vi "Single IV and Ic distribution v2.vi"() -> ()   [LabVIEW 2024]
uses:
  <vilib>/LabVIEW Targets/FPGA/cRIO/shared/nicrio_ModuleControls/nicrio_cRIO-9775_RecordDataRates4ChansRing.ctl
  RT fast data.ctl
  <vilib>/LabVIEW Targets/FPGA/cRIO/shared/nicrio_ModuleControls/nicrio_BasicConversionTime.ctl
  Ramps.ctl
  cRIO VI parameters.vi
  <resource>/objmgr/ni.dex.rc
  <vilib>/Analysis/NI_AALBase.lvlib
panel:
  in  "Tab Control 3":enum32{"Distribution", "IV"}(tab)
  out "Histogram Graph":T1(graph)={"X Values"=[3.702567138671875, 3.708775634765625, 3.714984130859375, 3.7211926269531252, 3.7274011230468753, 3.7336096191406254, 3.7398181152343755, 3.7460266113281255, 3.7522351074218756, 3.7584436035156257, 3.7646520996093757, 3.770860595703126, 3.777069091796876, 3.783277587890626, 3.789486083984376, 3.795694580078126, 3.801903076171876, 3.8081115722656262, 3.8143200683593763, 3.8205285644531264, 3.8267370605468765, 3.8329455566406265, 3.8391540527343766, 3.8453625488281267, 3.8515710449218767, 3.857779541015627, 3.863988037109377, 3.870196533203127, 3.876405029296877, 3.882613525390627, 3.888822021484377, 3.8950305175781272, 3.9012390136718773, 3.9074475097656274, 3.9136560058593775, 3.9198645019531275, 3.9260729980468776, 3.9322814941406277, 3.9384899902343777, 3.944698486328128, 3.950906982421878, 3.957115478515628, 3.963323974609378, 3.969532470703128, 3.975740966796878, 3.9819494628906282, 3.9881579589843783, 3.9943664550781284, 4.0005749511718784, 4.0067834472656285, 4.012991943359379, 4.019200439453129, 4.025408935546879, 4.031617431640629, 4.037825927734379, 4.044034423828129, 4.050242919921879, 4.056451416015629, 4.062659912109379, 4.068868408203129, 4.075076904296879, 4.081285400390629, 4.087493896484379, 4.0937023925781295, 4.09991088867188, 4.10611938476563, 4.11232788085938, 4.11853637695313, 4.12474487304688, 4.13095336914063, 4.13716186523438, 4.14337036132813, 4.14957885742188, 4.15578735351563, 4.16199584960938, 4.16820434570313, 4.17441284179688, 4.1806213378906305, 4.186829833984381, 4.193038330078131, 4.199246826171881, 4.205455322265631, 4.211663818359381, 4.217872314453131, 4.224080810546881, 4.230289306640631, 4.236497802734381, 4.242706298828131, 4.248914794921881, 4.255123291015631, 4.261331787109381, 4.2675402832031315, 4.273748779296882, 4.279957275390632, 4.286165771484382, 4.292374267578132, 4.298582763671882, 4.304791259765632, 4.310999755859382, 4.317208251953132], "Histogram: h(x)"=[1, 0, 0, 0, 1, 1, 0, 3, 2, 4, 3, 2, 1, 5, 10, 11, 14, 19, 24, 21, 32, 20, 49, 60, 74, 75, 110, 85, 117, 114, 161, 127, 186, 168, 225, 211, 265, 245, 280, 241, 355, 309, 353, 285, 369, 286, 349, 271, 355, 304, 277, 301, 252, 286, 218, 288, 193, 251, 165, 214, 135, 154, 132, 137, 101, 120, 75, 86, 58, 75, 49, 45, 25, 29, 25, 12, 20, 11, 9, 13, 5, 6, 4, 7, 2, 6, 1, 2, 1, 0, 1, 2, 1, 1, 0, 0, 0, 0, 1, 1]}
  out "Array":dbl[](array[numeric])
  out "Start time ms":u32=3399600001
  out "Time to Init ms":u32=668
  out "Threshold":dbl=0.23218066406250001
  out "IV Curve":cluster{"X":dbl[], "Y":dbl[]}[](graph)
  in  "length":i32=3300
  in  "Begin index":i32
  out "I data":dbl[](array[numeric])
  in  "Tab Control":T2(tab)
  in  "Data folder":path=path "C:/Users/gyue/Desktop/GA01_202401"
  in  "Sample Name":string
  out "output file name":string="20240127-224058-Single IV and Dist_Dist.dat"
  in  "IV Record Samples":u32=4300
  in  "Dist Records Num":i32=10000
  in  "IV Record Data Rate":T3=200 items=["20.000 MS/s (NI 9775)"=1, "10.00 MS/s (NI 9775)"=2, "6.667 MS/s (NI 9775)"=3, "5.000 MS/s (NI 9775)"=4, "2.500 MS/s (NI 9775)"=8, "1.667 MS/s (NI 9775)"=12, "1.250 MS/s (NI 9775)"=16, "1.000 MS/s (NI 9775)"=20, "833.333 KS/s (NI 9775)"=24, "714.286 KS/s (NI 9775)"=28, "625.000 KS/s (NI 9775)"=32, "555.556 KS/s (NI 9775)"=36, "500.000 KS/s (NI 9775)"=40, "454.545 KS/s (NI 9775)"=44, "416.667 KS/s (NI 9775)"=48, "384.615 KS/s (NI 9775)"=52, "357.143 KS/s (NI 9775)"=56, "333.333 KS/s (NI 9775)"=60, "312.500 KS/s (NI 9775)"=64, "294.118 KS/s (NI 9775)"=68, "277.778 KS/s (NI 9775)"=72, "263.158 KS/s (NI 9775)"=76, "250.000 KS/s (NI 9775)"=80, "238.095 KS/s (NI 9775)"=84, "227.273 KS/s (NI 9775)"=88, "217.391 KS/s (NI 9775)"=92, "208.333 KS/s (NI 9775)"=96, "200.000 KS/s (NI 9775)"=100, "192.308 KS/s (NI 9775)"=104, "185.185 KS/s (NI 9775)"=108, "178.571 KS/s (NI 9775)"=112, "172.414 KS/s (NI 9775)"=116, "166.667 KS/s (NI 9775)"=120, "161.290 KS/s (NI 9775)"=124, "156.250 KS/s (NI 9775)"=128, "151.515 KS/s (NI 9775)"=132, "147.059 KS/s (NI 9775)"=136, "142.857 KS/s (NI 9775)"=140, "138.889 KS/s (NI 9775)"=144, "135.135 KS/s (NI 9775)"=148, "131.579 KS/s (NI 9775)"=152, "128.205 KS/s (NI 9775)"=156, "125.000 KS/s (NI 9775)"=160, "121.951 KS/s (NI 9775)"=164, "119.048 KS/s (NI 9775)"=168, "116.279 KS/s (NI 9775)"=172, "113.636 KS/s (NI 9775)"=176, "111.111 KS/s (NI 9775)"=180, "108.696 KS/s (NI 9775)"=184, "106.383 KS/s (NI 9775)"=188, "104.167 KS/s (NI 9775)"=192, "102.041 KS/s (NI 9775)"=196, "100.000 KS/s (NI 9775)"=200, "50.000 KS/s (NI 9775)"=400, "33.333 KS/s (NI 9775)"=600, "25.000 KS/s (NI 9775)"=800, "20.000 KS/s (NI 9775)"=1000, "16.667 KS/s (NI 9775)"=1200, "14.286 KS/s (NI 9775)"=1400, "12.500 KS/s (NI 9775)"=1600, "11.111 KS/s (NI 9775)"=1800, "10.000 KS/s (NI 9775)"=2000, "9.091 KS/s (NI 9775)"=2200, "8.333 KS/s (NI 9775)"=2400, "7.692 KS/s (NI 9775)"=2600, "7.143 KS/s (NI 9775)"=2800, "6.667 KS/s (NI 9775)"=3000, "6.250 KS/s (NI 9775)"=3200, "5.882 KS/s (NI 9775)"=3400, "5.556 KS/s (NI 9775)"=3600, "5.000 KS/s (NI 9775)"=4000, "4.762 KS/s (NI 9775)"=4200, "4.545 KS/s (NI 9775)"=4400, "4.348 KS/s (NI 9775)"=4600, "4.167 KS/s (NI 9775)"=4800, "4.000 KS/s (NI 9775)"=5000, "3.846 KS/s (NI 9775)"=5200, "3.571 KS/s (NI 9775)"=5600, "3.333 KS/s (NI 9775)"=6000, "3.125 KS/s (NI 9775)"=6400, "2.941 KS/s (NI 9775)"=6800, "2.778 KS/s (NI 9775)"=7200, "2.632 KS/s (NI 9775)"=7600, "2.500 KS/s (NI 9775)"=8000, "2.381 KS/s (NI 9775)"=8400, "2.273 KS/s (NI 9775)"=8800, "2.174 KS/s (NI 9775)"=9200, "2.083 KS/s (NI 9775)"=9600, "2.000 KS/s (NI 9775)"=10000, "1.923 KS/s (NI 9775)"=10400, "1.852 KS/s (NI 9775)"=10800, "1.786 KS/s (NI 9775)"=11200, "1.724 KS/s (NI 9775)"=11600, "1.667 KS/s (NI 9775)"=12000, "1.613 KS/s (NI 9775)"=12400, "1.563 KS/s (NI 9775)"=12800, "1.515 KS/s (NI 9775)"=13200, "1.471 KS/s (NI 9775)"=13600, "1.429 KS/s (NI 9775)"=14000, "1.389 KS/s (NI 9775)"=14400, "1.351 KS/s (NI 9775)"=14800, "1.316 KS/s (NI 9775)"=15200, "1.282 KS/s (NI 9775)"=15600, "1.250 KS/s (NI 9775)"=16000, "1.220 KS/s (NI 9775)"=16400, "1.190 KS/s (NI 9775)"=16800, "1.163 KS/s (NI 9775)"=17200, "1.136 KS/s (NI 9775)"=17600, "1.111 KS/s (NI 9775)"=18000, "1.087 KS/s (NI 9775)"=18400, "1.064 KS/s (NI 9775)"=18800, "1.042 KS/s (NI 9775)"=19200, "1.020 KS/s (NI 9775)"=19600, "1.000 KS/s (NI 9775)"=20000, "0.980 KS/s (NI 9775)"=20400, "0.962 KS/s (NI 9775)"=20800, "0.943 KS/s (NI 9775)"=21200, "0.926 KS/s (NI 9775)"=21600, "0.909 KS/s (NI 9775)"=22000, "0.893 KS/s (NI 9775)"=22400, "0.877 KS/s (NI 9775)"=22800, "0.862 KS/s (NI 9775)"=23200, "0.847 KS/s (NI 9775)"=23600, "0.833 KS/s (NI 9775)"=24000, "0.820 KS/s (NI 9775)"=24400, "0.806 KS/s (NI 9775)"=24800, "0.794 KS/s (NI 9775)"=25200, "0.781 KS/s (NI 9775)"=25600, "0.694 KS/s (NI 9775)"=28800, "0.625 KS/s (NI 9775)"=32000, "0.568 KS/s (NI 9775)"=35200, "0.521 KS/s (NI 9775)"=38400, "0.446 KS/s (NI 9775)"=44800, "0.391 KS/s (NI 9775)"=51200, "0.347 KS/s (NI 9775)"=57600, "0.313 KS/s (NI 9775)"=64000]
  in  "Current Scale factor":dbl=1.0
  in  "Voltage Scale factor":dbl=0.0001
  in  "Relative Threshold":dbl=0.2
  in  "Read point":i32=1
  in  "Wire resistance":dbl
  in  "Zero avg":i32=1000
  in  "Ic Wait before trigger us":u32=30000
  in  "Ic Cutoff delay usec":u32
  in  "Trigger Slope":u16(ring) items=["Positive", "Negative"]
  in  "Tab Control 2":enum32{"IV parameters", "Ic parameters"}(tab)
  out "IV parameters":T4={"Records Num"=1, "AI Trigger Configuration"={"Trigger Slope"=enum."Positive", "Trigger Level"=0.10009765625, "Hystesis Value"=0.094970703125, "AI Channel"=0}, "Record PreTrigger Samples"=1, "Record Samples"=4300, "Ic Cut off or curve"=FALSE, "Record Data Rate"=200, "Wait before trigger us"=0, "Cutoff delay usec"=0, "Timing Mode"=enum."High Resolution", "Trigger length ticks"=1, "Timeout"=-1, "Ramps"={"Amp"=8.0, "Delay time 10us"=3000, "Ramp1 time 10us"=1000, "Ramp2 time 10us"=200, "Ramp3 time 10us"=100, "End time 10us"=0}} {"Record Data Rate" items=["20.000 MS/s (NI 9775)"=1, "10.00 MS/s (NI 9775)"=2, "6.667 MS/s (NI 9775)"=3, "5.000 MS/s (NI 9775)"=4, "2.500 MS/s (NI 9775)"=8, "1.667 MS/s (NI 9775)"=12, "1.250 MS/s (NI 9775)"=16, "1.000 MS/s (NI 9775)"=20, "833.333 KS/s (NI 9775)"=24, "714.286 KS/s (NI 9775)"=28, "625.000 KS/s (NI 9775)"=32, "555.556 KS/s (NI 9775)"=36, "500.000 KS/s (NI 9775)"=40, "454.545 KS/s (NI 9775)"=44, "416.667 KS/s (NI 9775)"=48, "384.615 KS/s (NI 9775)"=52, "357.143 KS/s (NI 9775)"=56, "333.333 KS/s (NI 9775)"=60, "312.500 KS/s (NI 9775)"=64, "294.118 KS/s (NI 9775)"=68, "277.778 KS/s (NI 9775)"=72, "263.158 KS/s (NI 9775)"=76, "250.000 KS/s (NI 9775)"=80, "238.095 KS/s (NI 9775)"=84, "227.273 KS/s (NI 9775)"=88, "217.391 KS/s (NI 9775)"=92, "208.333 KS/s (NI 9775)"=96, "200.000 KS/s (NI 9775)"=100, "192.308 KS/s (NI 9775)"=104, "185.185 KS/s (NI 9775)"=108, "178.571 KS/s (NI 9775)"=112, "172.414 KS/s (NI 9775)"=116, "166.667 KS/s (NI 9775)"=120, "161.290 KS/s (NI 9775)"=124, "156.250 KS/s (NI 9775)"=128, "151.515 KS/s (NI 9775)"=132, "147.059 KS/s (NI 9775)"=136, "142.857 KS/s (NI 9775)"=140, "138.889 KS/s (NI 9775)"=144, "135.135 KS/s (NI 9775)"=148, "131.579 KS/s (NI 9775)"=152, "128.205 KS/s (NI 9775)"=156, "125.000 KS/s (NI 9775)"=160, "121.951 KS/s (NI 9775)"=164, "119.048 KS/s (NI 9775)"=168, "116.279 KS/s (NI 9775)"=172, "113.636 KS/s (NI 9775)"=176, "111.111 KS/s (NI 9775)"=180, "108.696 KS/s (NI 9775)"=184, "106.383 KS/s (NI 9775)"=188, "104.167 KS/s (NI 9775)"=192, "102.041 KS/s (NI 9775)"=196, "100.000 KS/s (NI 9775)"=200, "50.000 KS/s (NI 9775)"=400, "33.333 KS/s (NI 9775)"=600, "25.000 KS/s (NI 9775)"=800, "20.000 KS/s (NI 9775)"=1000, "16.667 KS/s (NI 9775)"=1200, "14.286 KS/s (NI 9775)"=1400, "12.500 KS/s (NI 9775)"=1600, "11.111 KS/s (NI 9775)"=1800, "10.000 KS/s (NI 9775)"=2000, "9.091 KS/s (NI 9775)"=2200, "8.333 KS/s (NI 9775)"=2400, "7.692 KS/s (NI 9775)"=2600, "7.143 KS/s (NI 9775)"=2800, "6.667 KS/s (NI 9775)"=3000, "6.250 KS/s (NI 9775)"=3200, "5.882 KS/s (NI 9775)"=3400, "5.556 KS/s (NI 9775)"=3600, "5.000 KS/s (NI 9775)"=4000, "4.762 KS/s (NI 9775)"=4200, "4.545 KS/s (NI 9775)"=4400, "4.348 KS/s (NI 9775)"=4600, "4.167 KS/s (NI 9775)"=4800, "4.000 KS/s (NI 9775)"=5000, "3.846 KS/s (NI 9775)"=5200, "3.571 KS/s (NI 9775)"=5600, "3.333 KS/s (NI 9775)"=6000, "3.125 KS/s (NI 9775)"=6400, "2.941 KS/s (NI 9775)"=6800, "2.778 KS/s (NI 9775)"=7200, "2.632 KS/s (NI 9775)"=7600, "2.500 KS/s (NI 9775)"=8000, "2.381 KS/s (NI 9775)"=8400, "2.273 KS/s (NI 9775)"=8800, "2.174 KS/s (NI 9775)"=9200, "2.083 KS/s (NI 9775)"=9600, "2.000 KS/s (NI 9775)"=10000, "1.923 KS/s (NI 9775)"=10400, "1.852 KS/s (NI 9775)"=10800, "1.786 KS/s (NI 9775)"=11200, "1.724 KS/s (NI 9775)"=11600, "1.667 KS/s (NI 9775)"=12000, "1.613 KS/s (NI 9775)"=12400, "1.563 KS/s (NI 9775)"=12800, "1.515 KS/s (NI 9775)"=13200, "1.471 KS/s (NI 9775)"=13600, "1.429 KS/s (NI 9775)"=14000, "1.389 KS/s (NI 9775)"=14400, "1.351 KS/s (NI 9775)"=14800, "1.316 KS/s (NI 9775)"=15200, "1.282 KS/s (NI 9775)"=15600, "1.250 KS/s (NI 9775)"=16000, "1.220 KS/s (NI 9775)"=16400, "1.190 KS/s (NI 9775)"=16800, "1.163 KS/s (NI 9775)"=17200, "1.136 KS/s (NI 9775)"=17600, "1.111 KS/s (NI 9775)"=18000, "1.087 KS/s (NI 9775)"=18400, "1.064 KS/s (NI 9775)"=18800, "1.042 KS/s (NI 9775)"=19200, "1.020 KS/s (NI 9775)"=19600, "1.000 KS/s (NI 9775)"=20000, "0.980 KS/s (NI 9775)"=20400, "0.962 KS/s (NI 9775)"=20800, "0.943 KS/s (NI 9775)"=21200, "0.926 KS/s (NI 9775)"=21600, "0.909 KS/s (NI 9775)"=22000, "0.893 KS/s (NI 9775)"=22400, "0.877 KS/s (NI 9775)"=22800, "0.862 KS/s (NI 9775)"=23200, "0.847 KS/s (NI 9775)"=23600, "0.833 KS/s (NI 9775)"=24000, "0.820 KS/s (NI 9775)"=24400, "0.806 KS/s (NI 9775)"=24800, "0.794 KS/s (NI 9775)"=25200, "0.781 KS/s (NI 9775)"=25600, "0.694 KS/s (NI 9775)"=28800, "0.625 KS/s (NI 9775)"=32000, "0.568 KS/s (NI 9775)"=35200, "0.521 KS/s (NI 9775)"=38400, "0.446 KS/s (NI 9775)"=44800, "0.391 KS/s (NI 9775)"=51200, "0.347 KS/s (NI 9775)"=57600, "0.313 KS/s (NI 9775)"=64000]}
  out "Ic parameters":T4={"Records Num"=10000, "AI Trigger Configuration"={"Trigger Slope"=enum."Positive", "Trigger Level"=0.232177734375, "Hystesis Value"=0.0, "AI Channel"=0}, "Record PreTrigger Samples"=1, "Record Samples"=16, "Ic Cut off or curve"=TRUE, "Record Data Rate"=1, "Wait before trigger us"=30000, "Cutoff delay usec"=0, "Timing Mode"=enum."High Resolution", "Trigger length ticks"=1, "Timeout"=-1, "Ramps"={"Amp"=8.0, "Delay time 10us"=3000, "Ramp1 time 10us"=1000, "Ramp2 time 10us"=200, "Ramp3 time 10us"=100, "End time 10us"=0}} {"Record Data Rate" items=["20.000 MS/s (NI 9775)"=1, "10.00 MS/s (NI 9775)"=2, "6.667 MS/s (NI 9775)"=3, "5.000 MS/s (NI 9775)"=4, "2.500 MS/s (NI 9775)"=8, "1.667 MS/s (NI 9775)"=12, "1.250 MS/s (NI 9775)"=16, "1.000 MS/s (NI 9775)"=20, "833.333 KS/s (NI 9775)"=24, "714.286 KS/s (NI 9775)"=28, "625.000 KS/s (NI 9775)"=32, "555.556 KS/s (NI 9775)"=36, "500.000 KS/s (NI 9775)"=40, "454.545 KS/s (NI 9775)"=44, "416.667 KS/s (NI 9775)"=48, "384.615 KS/s (NI 9775)"=52, "357.143 KS/s (NI 9775)"=56, "333.333 KS/s (NI 9775)"=60, "312.500 KS/s (NI 9775)"=64, "294.118 KS/s (NI 9775)"=68, "277.778 KS/s (NI 9775)"=72, "263.158 KS/s (NI 9775)"=76, "250.000 KS/s (NI 9775)"=80, "238.095 KS/s (NI 9775)"=84, "227.273 KS/s (NI 9775)"=88, "217.391 KS/s (NI 9775)"=92, "208.333 KS/s (NI 9775)"=96, "200.000 KS/s (NI 9775)"=100, "192.308 KS/s (NI 9775)"=104, "185.185 KS/s (NI 9775)"=108, "178.571 KS/s (NI 9775)"=112, "172.414 KS/s (NI 9775)"=116, "166.667 KS/s (NI 9775)"=120, "161.290 KS/s (NI 9775)"=124, "156.250 KS/s (NI 9775)"=128, "151.515 KS/s (NI 9775)"=132, "147.059 KS/s (NI 9775)"=136, "142.857 KS/s (NI 9775)"=140, "138.889 KS/s (NI 9775)"=144, "135.135 KS/s (NI 9775)"=148, "131.579 KS/s (NI 9775)"=152, "128.205 KS/s (NI 9775)"=156, "125.000 KS/s (NI 9775)"=160, "121.951 KS/s (NI 9775)"=164, "119.048 KS/s (NI 9775)"=168, "116.279 KS/s (NI 9775)"=172, "113.636 KS/s (NI 9775)"=176, "111.111 KS/s (NI 9775)"=180, "108.696 KS/s (NI 9775)"=184, "106.383 KS/s (NI 9775)"=188, "104.167 KS/s (NI 9775)"=192, "102.041 KS/s (NI 9775)"=196, "100.000 KS/s (NI 9775)"=200, "50.000 KS/s (NI 9775)"=400, "33.333 KS/s (NI 9775)"=600, "25.000 KS/s (NI 9775)"=800, "20.000 KS/s (NI 9775)"=1000, "16.667 KS/s (NI 9775)"=1200, "14.286 KS/s (NI 9775)"=1400, "12.500 KS/s (NI 9775)"=1600, "11.111 KS/s (NI 9775)"=1800, "10.000 KS/s (NI 9775)"=2000, "9.091 KS/s (NI 9775)"=2200, "8.333 KS/s (NI 9775)"=2400, "7.692 KS/s (NI 9775)"=2600, "7.143 KS/s (NI 9775)"=2800, "6.667 KS/s (NI 9775)"=3000, "6.250 KS/s (NI 9775)"=3200, "5.882 KS/s (NI 9775)"=3400, "5.556 KS/s (NI 9775)"=3600, "5.000 KS/s (NI 9775)"=4000, "4.762 KS/s (NI 9775)"=4200, "4.545 KS/s (NI 9775)"=4400, "4.348 KS/s (NI 9775)"=4600, "4.167 KS/s (NI 9775)"=4800, "4.000 KS/s (NI 9775)"=5000, "3.846 KS/s (NI 9775)"=5200, "3.571 KS/s (NI 9775)"=5600, "3.333 KS/s (NI 9775)"=6000, "3.125 KS/s (NI 9775)"=6400, "2.941 KS/s (NI 9775)"=6800, "2.778 KS/s (NI 9775)"=7200, "2.632 KS/s (NI 9775)"=7600, "2.500 KS/s (NI 9775)"=8000, "2.381 KS/s (NI 9775)"=8400, "2.273 KS/s (NI 9775)"=8800, "2.174 KS/s (NI 9775)"=9200, "2.083 KS/s (NI 9775)"=9600, "2.000 KS/s (NI 9775)"=10000, "1.923 KS/s (NI 9775)"=10400, "1.852 KS/s (NI 9775)"=10800, "1.786 KS/s (NI 9775)"=11200, "1.724 KS/s (NI 9775)"=11600, "1.667 KS/s (NI 9775)"=12000, "1.613 KS/s (NI 9775)"=12400, "1.563 KS/s (NI 9775)"=12800, "1.515 KS/s (NI 9775)"=13200, "1.471 KS/s (NI 9775)"=13600, "1.429 KS/s (NI 9775)"=14000, "1.389 KS/s (NI 9775)"=14400, "1.351 KS/s (NI 9775)"=14800, "1.316 KS/s (NI 9775)"=15200, "1.282 KS/s (NI 9775)"=15600, "1.250 KS/s (NI 9775)"=16000, "1.220 KS/s (NI 9775)"=16400, "1.190 KS/s (NI 9775)"=16800, "1.163 KS/s (NI 9775)"=17200, "1.136 KS/s (NI 9775)"=17600, "1.111 KS/s (NI 9775)"=18000, "1.087 KS/s (NI 9775)"=18400, "1.064 KS/s (NI 9775)"=18800, "1.042 KS/s (NI 9775)"=19200, "1.020 KS/s (NI 9775)"=19600, "1.000 KS/s (NI 9775)"=20000, "0.980 KS/s (NI 9775)"=20400, "0.962 KS/s (NI 9775)"=20800, "0.943 KS/s (NI 9775)"=21200, "0.926 KS/s (NI 9775)"=21600, "0.909 KS/s (NI 9775)"=22000, "0.893 KS/s (NI 9775)"=22400, "0.877 KS/s (NI 9775)"=22800, "0.862 KS/s (NI 9775)"=23200, "0.847 KS/s (NI 9775)"=23600, "0.833 KS/s (NI 9775)"=24000, "0.820 KS/s (NI 9775)"=24400, "0.806 KS/s (NI 9775)"=24800, "0.794 KS/s (NI 9775)"=25200, "0.781 KS/s (NI 9775)"=25600, "0.694 KS/s (NI 9775)"=28800, "0.625 KS/s (NI 9775)"=32000, "0.568 KS/s (NI 9775)"=35200, "0.521 KS/s (NI 9775)"=38400, "0.446 KS/s (NI 9775)"=44800, "0.391 KS/s (NI 9775)"=51200, "0.347 KS/s (NI 9775)"=57600, "0.313 KS/s (NI 9775)"=64000]}
  out "Ramps Cluster":T6={"Amp"=8.0, "Delay time 10us"=3000, "Ramp1 time 10us"=1000, "Ramp2 time 10us"=200, "Ramp3 time 10us"=100, "End time 10us"=0}
  in  "Amp":dbl=8.0
  in  "Delay time 10us":i32=3000
  in  "Ramp1 time 10us":i32=1000
  in  "Ramp2 time 10us":i32=200
  in  "Ramp3 time 10us":i32=100
  in  "End time 10us":i32
  out "DAQ_CMD_Writer endpoint":refnum<k21>="DAQ_CMD_Writer"
  out "DAQ_AI_Reader endpoint":refnum<k21>="DAQ_AI_Reader"
  out "PCreaderI":refnum<k21>="PCreaderI"
  out "PC para writer":refnum<k21>="PCwriter"
  out "PCreaderV":refnum<k21>="PCreaderV"
  out "error out":errorcluster
  out "Done":bool=TRUE
  # "Voltage x factor=uA"
  # "Voltage x factor=actual Volt"
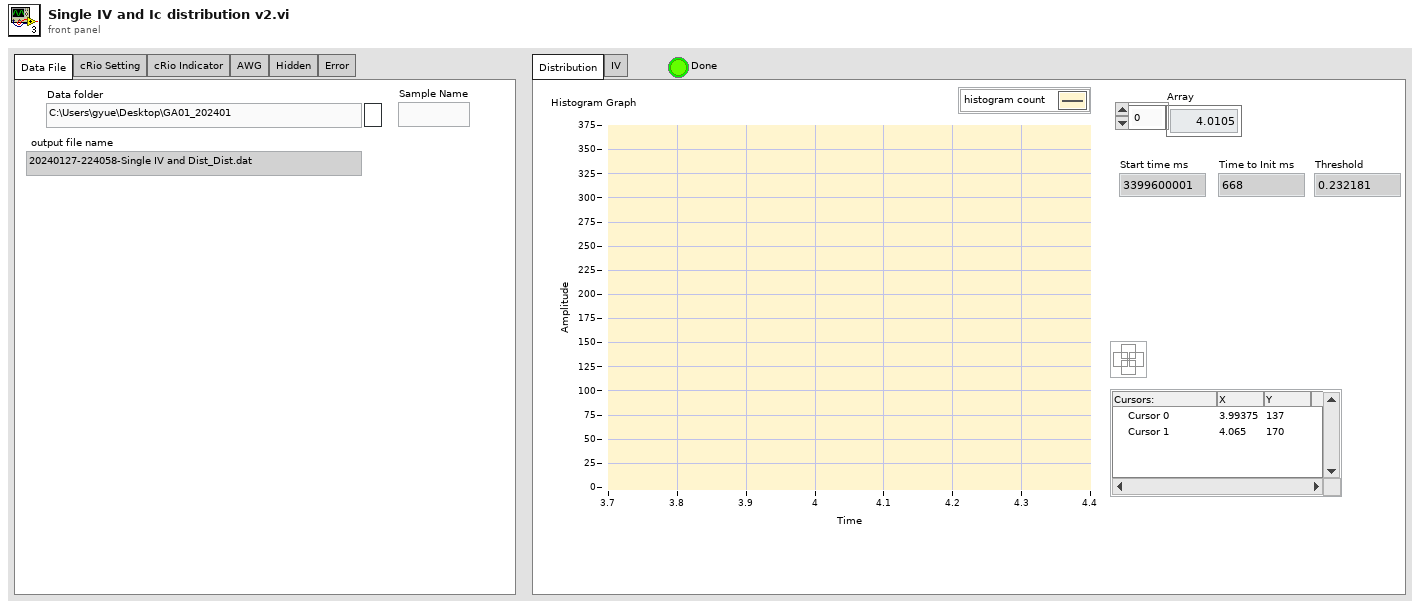
[diagram p1: front panel]
types:
  T1 = cluster{"X Values":dbl[], "Histogram: h(x)":i32[]}
  T2 = enum32{"Data File", "cRio Setting", "cRio Indicator", "AWG", "Hidden", "Error"}
  T3 = typedef "nicrio_cRIO-9775_RecordDataRates4ChansRing.ctl" = u16
  T4 = typedef "RT fast data.ctl" = cluster{"Records Num":i32, "AI Trigger Configuration":cluster{"Trigger Slope":enum8{"Positive", "Negative"}, "Trigger Level":fxp<+/-,17,5>, "Hystesis Value":fxp<+,16,4>, "AI Channel":u8}, "Record PreTrigger Samples":u32, "Record Samples":u32, "Ic Cut off or curve":bool, "Record Data Rate":T3, "Wait before trigger us":u32, "Cutoff delay usec":u32, "Timing Mode":T5, "Trigger length ticks":u32, "Timeout":i32, "Ramps":T6}
  T5 = typedef "nicrio_BasicConversionTime.ctl" = enum8{"High Speed", "High Resolution"}
  T6 = typedef "Ramps.ctl" = cluster{"Amp":fxp<+/-,20,5>, "Delay time 10us":i32, "Ramp1 time 10us":i32, "Ramp2 time 10us":i32, "Ramp3 time 10us":i32, "End time 10us":i32}
  T7 = cluster{"Trigger Slope":enum8{"Positive", "Negative"}, "Trigger Level":fxp<+/-,17,5>, "Hystesis Value":fxp<+,16,4>, "AI Channel":u8}
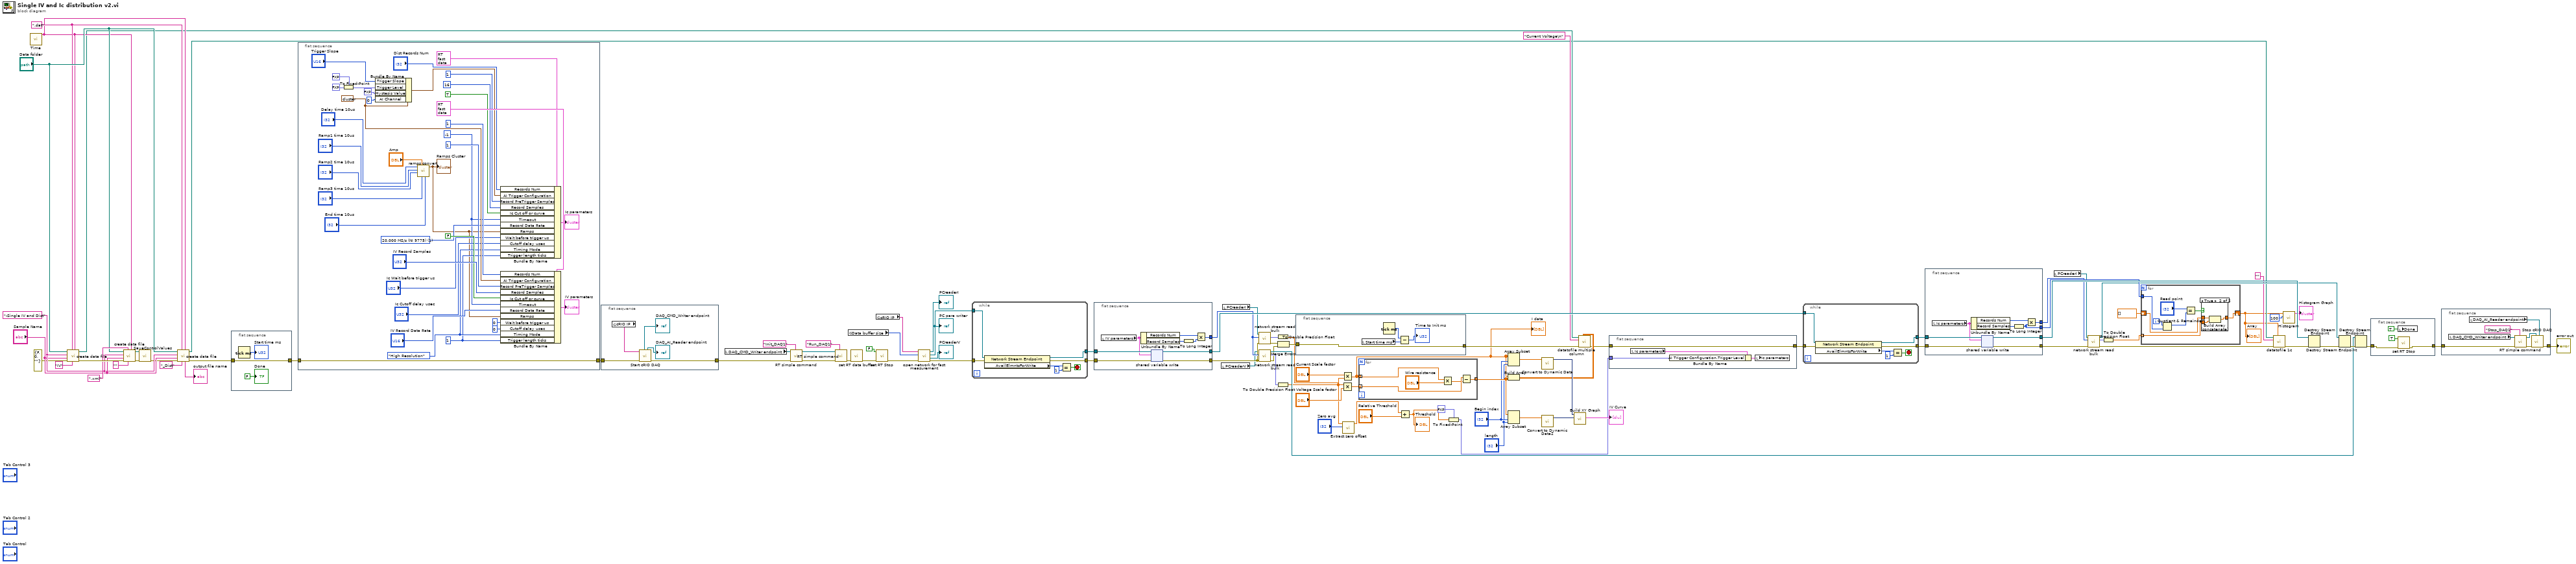
[diagram p0: block diagram]
diagram:
  w59 = ".dat" ("Ext name")
  w61 = "-Single IV and Dist" ("Measurement Name")
  n1 = call "Time.vi"() -> ("Timestamp"=w58:string)  [unwired: 11 in]
  n2 = call "create data file.vi"("Time"=w58, "end string"="IV", "Ext name"=w59, "error in (no error)"=errorcluster {"status"=FALSE, "code"=0, "source"=""}, "Sample Name"="Sample Name", "Measurement Name"=w61, "base path"="Data folder") -> ("error out"=w67:errorcluster, "appended path"=w57:path)  [unwired: 2 in, 1 out]
  n3 = call "create data file.vi"("Time"=w58, "end string"="", "Ext name"=".xml", "error in (no error)"=w67, "Sample Name"="Sample Name", "Measurement Name"=w61, "base path"="Data folder") -> ("error out"=w46:errorcluster, "appended path"=w47:path)  [unwired: 2 in, 1 out]
  n4 = call "SaveControlValues.vi"("XML File Path"=w47, "error in (no error)"=w46) -> ("error out"=w45:errorcluster)  [unwired: 8 in]
  n5 = call "create data file.vi"("Time"=w58, "end string"="_Dist", "Ext name"=w59, "error in (no error)"=w45, "Sample Name"="Sample Name", "Measurement Name"=w61, "base path"="Data folder") -> ("error out"=w64:errorcluster, "appended path"=w53:path, "file name"=→"output file name":string)  [unwired: 2 in]
  n6 = flat-sequence {
    tunnel: [w98] -> w44
    tunnel: w64 -> [w98]
    frame #0 {
      n7 = Tick Count (ms)() -> (millisecond timer value=→"Start time ms":u32)
      "Done" <- FALSE ("Done")
    }
  }
  n8 = flat-sequence {
    tunnel: w44 -> [w129]
    tunnel: [w129] -> w23
    frame #0 {
      w109 = -1 ("Timeout")
      w110 = u32 1 ("Trigger length ticks")
      w111 = nicrio_BasicConversionTime."High Resolution" ("Timing Mode")
      w116 = T3 1 items=["20.000 MS/s (NI 9775)"=1, "10.00 MS/s (NI 9775)"=2, "6.667 MS/s (NI 9775)"=3, "5.000 MS/s (NI 9775)"=4, "2.500 MS/s (NI 9775)"=8, "1.667 MS/s (NI 9775)"=12, "1.250 MS/s (NI 9775)"=16, "1.000 MS/s (NI 9775)"=20, "833.333 KS/s (NI 9775)"=24, "714.286 KS/s (NI 9775)"=28, "625.000 KS/s (NI 9775)"=32, "555.556 KS/s (NI 9775)"=36, "500.000 KS/s (NI 9775)"=40, "454.545 KS/s (NI 9775)"=44, "416.667 KS/s (NI 9775)"=48, "384.615 KS/s (NI 9775)"=52, "357.143 KS/s (NI 9775)"=56, "333.333 KS/s (NI 9775)"=60, "312.500 KS/s (NI 9775)"=64, "294.118 KS/s (NI 9775)"=68, "277.778 KS/s (NI 9775)"=72, "263.158 KS/s (NI 9775)"=76, "250.000 KS/s (NI 9775)"=80, "238.095 KS/s (NI 9775)"=84, "227.273 KS/s (NI 9775)"=88, "217.391 KS/s (NI 9775)"=92, "208.333 KS/s (NI 9775)"=96, "200.000 KS/s (NI 9775)"=100, "192.308 KS/s (NI 9775)"=104, "185.185 KS/s (NI 9775)"=108, "178.571 KS/s (NI 9775)"=112, "172.414 KS/s (NI 9775)"=116, "166.667 KS/s (NI 9775)"=120, "161.290 KS/s (NI 9775)"=124, "156.250 KS/s (NI 9775)"=128, "151.515 KS/s (NI 9775)"=132, "147.059 KS/s (NI 9775)"=136, "142.857 KS/s (NI 9775)"=140, "138.889 KS/s (NI 9775)"=144, "135.135 KS/s (NI 9775)"=148, "131.579 KS/s (NI 9775)"=152, "128.205 KS/s (NI 9775)"=156, "125.000 KS/s (NI 9775)"=160, "121.951 KS/s (NI 9775)"=164, "119.048 KS/s (NI 9775)"=168, "116.279 KS/s (NI 9775)"=172, "113.636 KS/s (NI 9775)"=176, "111.111 KS/s (NI 9775)"=180, "108.696 KS/s (NI 9775)"=184, "106.383 KS/s (NI 9775)"=188, "104.167 KS/s (NI 9775)"=192, "102.041 KS/s (NI 9775)"=196, "100.000 KS/s (NI 9775)"=200, "50.000 KS/s (NI 9775)"=400, "33.333 KS/s (NI 9775)"=600, "25.000 KS/s (NI 9775)"=800, "20.000 KS/s (NI 9775)"=1000, "16.667 KS/s (NI 9775)"=1200, "14.286 KS/s (NI 9775)"=1400, "12.500 KS/s (NI 9775)"=1600, "11.111 KS/s (NI 9775)"=1800, "10.000 KS/s (NI 9775)"=2000, "9.091 KS/s (NI 9775)"=2200, "8.333 KS/s (NI 9775)"=2400, "7.692 KS/s (NI 9775)"=2600, "7.143 KS/s (NI 9775)"=2800, "6.667 KS/s (NI 9775)"=3000, "6.250 KS/s (NI 9775)"=3200, "5.882 KS/s (NI 9775)"=3400, "5.556 KS/s (NI 9775)"=3600, "5.000 KS/s (NI 9775)"=4000, "4.762 KS/s (NI 9775)"=4200, "4.545 KS/s (NI 9775)"=4400, "4.348 KS/s (NI 9775)"=4600, "4.167 KS/s (NI 9775)"=4800, "4.000 KS/s (NI 9775)"=5000, "3.846 KS/s (NI 9775)"=5200, "3.571 KS/s (NI 9775)"=5600, "3.333 KS/s (NI 9775)"=6000, "3.125 KS/s (NI 9775)"=6400, "2.941 KS/s (NI 9775)"=6800, "2.778 KS/s (NI 9775)"=7200, "2.632 KS/s (NI 9775)"=7600, "2.500 KS/s (NI 9775)"=8000, "2.381 KS/s (NI 9775)"=8400, "2.273 KS/s (NI 9775)"=8800, "2.174 KS/s (NI 9775)"=9200, "2.083 KS/s (NI 9775)"=9600, "2.000 KS/s (NI 9775)"=10000, "1.923 KS/s (NI 9775)"=10400, "1.852 KS/s (NI 9775)"=10800, "1.786 KS/s (NI 9775)"=11200, "1.724 KS/s (NI 9775)"=11600, "1.667 KS/s (NI 9775)"=12000, "1.613 KS/s (NI 9775)"=12400, "1.563 KS/s (NI 9775)"=12800, "1.515 KS/s (NI 9775)"=13200, "1.471 KS/s (NI 9775)"=13600, "1.429 KS/s (NI 9775)"=14000, "1.389 KS/s (NI 9775)"=14400, "1.351 KS/s (NI 9775)"=14800, "1.316 KS/s (NI 9775)"=15200, "1.282 KS/s (NI 9775)"=15600, "1.250 KS/s (NI 9775)"=16000, "1.220 KS/s (NI 9775)"=16400, "1.190 KS/s (NI 9775)"=16800, "1.163 KS/s (NI 9775)"=17200, "1.136 KS/s (NI 9775)"=17600, "1.111 KS/s (NI 9775)"=18000, "1.087 KS/s (NI 9775)"=18400, "1.064 KS/s (NI 9775)"=18800, "1.042 KS/s (NI 9775)"=19200, "1.020 KS/s (NI 9775)"=19600, "1.000 KS/s (NI 9775)"=20000, "0.980 KS/s (NI 9775)"=20400, "0.962 KS/s (NI 9775)"=20800, "0.943 KS/s (NI 9775)"=21200, "0.926 KS/s (NI 9775)"=21600, "0.909 KS/s (NI 9775)"=22000, "0.893 KS/s (NI 9775)"=22400, "0.877 KS/s (NI 9775)"=22800, "0.862 KS/s (NI 9775)"=23200, "0.847 KS/s (NI 9775)"=23600, "0.833 KS/s (NI 9775)"=24000, "0.820 KS/s (NI 9775)"=24400, "0.806 KS/s (NI 9775)"=24800, "0.794 KS/s (NI 9775)"=25200, "0.781 KS/s (NI 9775)"=25600, "0.694 KS/s (NI 9775)"=28800, "0.625 KS/s (NI 9775)"=32000, "0.568 KS/s (NI 9775)"=35200, "0.521 KS/s (NI 9775)"=38400, "0.446 KS/s (NI 9775)"=44800, "0.391 KS/s (NI 9775)"=51200, "0.347 KS/s (NI 9775)"=57600, "0.313 KS/s (NI 9775)"=64000] ("Record Data Rate")
      w124 = T7 {"Trigger Slope"=enum."Positive", "Trigger Level"=0.10009765625, "Hystesis Value"=0.094970703125, "AI Channel"=0} ("AI Trigger Configuration")
      n9 = To Fixed-Point(fixed-point type=fxp<+/-,17,5> 0.0 ("Trigger Level"), number=fxp<+/-,32,16> 0.0) -> (fixed-point=w121:fxp<+/-,17,5>)
      n10 = Bundle By Name(cluster=w124, "Trigger Slope"="Trigger Slope", "Trigger Level"=w121, "Hystesis Value"=fxp<+,16,4> 0.0, "AI Channel"=u8 0) -> (w118:T7)
      n11 = call "ramps convert.vi"("End time 10us"="End time 10us", "Ramp3 time 10us"="Ramp3 time 10us", "Amp"="Amp", "Ramp2 time 10us"="Ramp2 time 10us", "Ramp1 time 10us"="Ramp1 time 10us", "Delay time 10us"="Delay time 10us") -> ("Ramps cluster"=w102:T6)  [unwired: 5 in]
      "Ramps Cluster" <- w102
      n12 = Bundle By Name(cluster=T4 {"Records Num"=1, "AI Trigger Configuration"={"Trigger Slope"=enum."Positive", "Trigger Level"=0.10009765625, "Hystesis Value"=0.094970703125, "AI Channel"=0}, "Record PreTrigger Samples"=1, "Record Samples"=5000, "Ic Cut off or curve"=FALSE, "Record Data Rate"=200, "Wait before trigger us"=10100, "Cutoff delay usec"=500, "Timing Mode"=enum."High Resolution", "Trigger length ticks"=15, "Timeout"=-1, "Ramps"={"Amp"=0.0, "Delay time 10us"=1, "Ramp1 time 10us"=1000, "Ramp2 time 10us"=2000, "Ramp3 time 10us"=1000, "End time 10us"=1}} ("IV parameters 2"), "Records Num"="Dist Records Num", "AI Trigger Configuration"=w118, "Record PreTrigger Samples"=u32 1, "Record Samples"=u32 16, "Ic Cut off or curve"=TRUE, "Timeout"=w109, "Record Data Rate"=w116, "Ramps"=w102, "Wait before trigger us"="Ic Wait before trigger us", "Cutoff delay usec"="Ic Cutoff delay usec", "Timing Mode"=w111, "Trigger length ticks"=w110) -> (→"Ic parameters":T4)
      n13 = Bundle By Name(cluster=T4 {"Records Num"=1, "AI Trigger Configuration"={"Trigger Slope"=enum."Positive", "Trigger Level"=0.10009765625, "Hystesis Value"=0.094970703125, "AI Channel"=0}, "Record PreTrigger Samples"=1, "Record Samples"=5000, "Ic Cut off or curve"=FALSE, "Record Data Rate"=200, "Wait before trigger us"=10100, "Cutoff delay usec"=500, "Timing Mode"=enum."High Resolution", "Trigger length ticks"=15, "Timeout"=-1, "Ramps"={"Amp"=0.0, "Delay time 10us"=1, "Ramp1 time 10us"=1000, "Ramp2 time 10us"=2000, "Ramp3 time 10us"=1000, "End time 10us"=1}} ("IV parameters 2"), "Records Num"=1, "AI Trigger Configuration"=w124, "Record PreTrigger Samples"=u32 1, "Record Samples"="IV Record Samples", "Ic Cut off or curve"=FALSE, "Timeout"=w109, "Record Data Rate"="IV Record Data Rate", "Ramps"=w102, "Wait before trigger us"=u32 0, "Cutoff delay usec"=u32 0, "Timing Mode"=w111, "Trigger length ticks"=w110) -> (→"IV parameters":T4)
    }
  }
  n14 = flat-sequence {
    tunnel: w23 -> [w139]
    tunnel: [w138] -> w17
    frame #0 {
      n15 = global read "cRIO VI parameters.vi" "cRIO IP"() -> (w137:string)
      n16 = call "Start cRIO DAQ.vi"("error in (no error)"=w139, "cRIO IP"=w137) -> ("error out"=w138:errorcluster, "DAQ_AI_Reader endpoint"=→"DAQ_AI_Reader endpoint":refnum<k21>, "DAQ_CMD_Writer endpoint"=→"DAQ_CMD_Writer endpoint":refnum<k21>)  [unwired: 7 in]
    }
  }
  n17 = local read "DAQ_CMD_Writer endpoint"() -> (w22:refnum<k21>)
  n18 = call "RT simple command.vi"("Command"="Init_DAQ1", "error in (no error)"=w17, "DAQ_CMD_Writer endpoint"=w22) -> ("error out"=w20:errorcluster, "DAQ_CMD_Writer endpoint out"=w19:refnum<k21>)  [unwired: 7 in]
  n19 = call "RT simple command.vi"("Command"="Run_DAQ1", "error in (no error)"=w20, "DAQ_CMD_Writer endpoint"=w19) -> ("error out"=w7:errorcluster)  [unwired: 7 in, 1 out]
  n20 = global read "cRIO VI parameters.vi" "Data buffer size"() -> (w2:i32)
  n21 = call "set RT data buffer.vi"("error in (no error)"=w7) -> ("error out"=w6:errorcluster)  [unwired: 10 in]
  n22 = global read "cRIO VI parameters.vi" "cRIO IP"() -> (w3:string)
  n23 = call "set RT Stop.vi"("error in (no error)"=w6, "RT Stop"=FALSE) -> ("error out"=w4:errorcluster)  [unwired: 9 in]
  n24 = call "open network for fast measurement.vi"("error in (no error)"=w4, "Data buffer size"=w2, "cRIO IP"=w3) -> ("error out"=w14:errorcluster, "PCreaderV"=→"PCreaderV":refnum<k21>, "PC para writer"=w13:refnum<k21>, "PCreaderI"=→"PCreaderI":refnum<k21>)  [unwired: 5 in]
  "PC para writer" <- w13
  n25 = while {
    tunnel: w13 -> [w148]
    tunnel: w14 -> [w147]
    tunnel: [w143] -> w96
    tunnel: [w142] -> w80
    stop <- w144 stop-if-true
    n26 = property class="Network Stream Endpoint"(reference=w148, error in=w147) -> (reference out=w143:refnum<k21>, error out=w142:errorcluster, "AvailElmntsForWrite"=w146:i32)
    n27 = Equal?(x=w146, y=1) -> (x = y?=w144:bool)
  }
  n28 = flat-sequence {
    tunnel: w96 -> [w157]
    tunnel: [w156] -> w92
    tunnel: w80 -> [w152]
    tunnel: [w151] -> w76
    tunnel: [w150] -> w68
    frame #0 {
      n29 = local read "IV parameters"() -> (w149:T4)
      n30 = Unbundle By Name(w149) -> ("Records Num"=w155:i32, "Record Samples"=w154:u32)
      n31 = shared-variable-write(w157, w152, w149) -> (w156:refnum<k21>, w150:errorcluster)  [unwired: 1 in, 1 out]
      n32 = To Long Integer(number=w154) -> (32bit integer=w153:i32)
      n33 = Multiply(x=w155, y=w153) -> (x*y=w151:i32)
    }
  }
  n34 = local read "PCreaderV"() -> (w11:refnum<k21>)
  n35 = local read "PCreaderI"() -> (w12:refnum<k21>)
  n36 = call "network stream read bulk.vi"("endpoint in"=w12, "Data num"=w76, "error in (no error)"=w68) -> ("Data"=w78:fxp<+/-,17,5>[], "error out"=w74:errorcluster)  [unwired: 5 in, 1 out]
  n37 = call "network stream read bulk.vi"("endpoint in"=w11, "Data num"=w76, "error in (no error)"=w68) -> ("endpoint out"=w75:refnum<k21>, "Data"=w77:fxp<+/-,17,5>[], "error out"=w73:errorcluster)  [unwired: 5 in]
  n38 = To Double Precision Float(number=w78) -> (double precision float=w42:dbl[])
  n39 = Merge Errors(w74, w73) -> (w79:errorcluster)
  n40 = To Double Precision Float(number=w77) -> (double precision float=w30:dbl[])
  n41 = flat-sequence {
    tunnel: w79 -> [w158]
    tunnel: [w158] -> w54
    frame #0 {
      n42 = local read "Start time ms"() -> (w160:u32)
      n43 = Tick Count (ms)() -> (millisecond timer value=w161:u32)
      n44 = Subtract(x=w161, y=w160) -> (x-y=→"Time to Init ms":u32)
    }
  }
  n45 = Multiply(x=w30, y="Voltage Scale factor") -> (x*y=w40:dbl[])
  n46 = Multiply(x="Current Scale factor", y=w42) -> (x*y=w1:dbl[])
  "I data" <- w1
  n47 = call "Extract zero offset.vi"("Zero avg num"="Zero avg", "Array"=w30) -> ("Offset"=w33:dbl)  [unwired: 9 in]
  n48 = for {
    tunnel: w40 -> [w166] mode=indexing
    tunnel: w1 -> [w164] mode=indexing
    tunnel: [w162] -> w38 mode=indexing
    n49 = Multiply(x=w164, y="Wire resistance") -> (x*y=w163:dbl)
    n50 = Subtract(x=w166, y=w163) -> (x-y=w162:dbl)
  }
  n51 = Add(x=w33, y="Relative Threshold") -> (x+y=w31:dbl)
  "Threshold" <- w31
  n52 = To Fixed-Point(fixed-point type=fxp<+,16,4> 0.0 ("AI Trigger Configuration.Hystesis Value"), number=w31) -> (fixed-point=w25:fxp<+,16,4>)
  n53 = Array Subset(array=w1, index="Begin index", length="length") -> (w39:dbl[])
  n54 = Build Array(w1, w38) -> (w55:dbl[][])
  n55 = Array Subset(array=w38, index="Begin index", length="length") -> (w37:dbl[])
  n56 = call "Convert to Dynamic Data"("Array"=w39) -> ("Dynamic Data Type"=w87:dynamicdata)  [unwired: 3 in]
  n57 = call "Convert to Dynamic Data2"("Array"=w37) -> ("Dynamic Data Type"=w86:dynamicdata)  [unwired: 3 in]
  n58 = call "Build XY Graph"("Y Input"=w86, "X Input"=w87) -> ("XY Graph"=→"IV Curve":cluster{"X":dbl[], "Y":dbl[]}[])  [unwired: 8 in, 1 out]
  n59 = call "datatofile multiple column.vi"("2D data"=w55, "error in"=w54, "title"="Current Voltage\n", "file path (dialog if empty)"=w57) -> ("error out"=w28:errorcluster)  [unwired: 7 in]
  n60 = flat-sequence {
    tunnel: w28 -> [w170]
    tunnel: [w170] -> w27
    tunnel: w25 -> [w169]
    frame #0 {
      n61 = local read "Ic parameters"() -> (w167:T4)
      n62 = Bundle By Name(cluster=w167, "AI Trigger Configuration.Trigger Level"=w169) -> (w168:T4)
      n63 = local write "Ic parameters"(w168) -> ()
    }
  }
  n64 = while {
    tunnel: w92 -> [w175]
    tunnel: w27 -> [w174]
    tunnel: [w172] -> w91
    tunnel: [w171] -> w90
    stop <- w173 stop-if-true
    n65 = property class="Network Stream Endpoint"(reference=w175, error in=w174) -> (reference out=w172:refnum<k21>, error out=w171:errorcluster, "AvailElmntsForWrite"=w177:i32)
    n66 = Equal?(x=w177, y=1) -> (x = y?=w173:bool)
  }
  n67 = flat-sequence {
    tunnel: w91 -> [w186]
    tunnel: w90 -> [w185]
    tunnel: [w184] -> w88
    tunnel: [w180] -> w82
    tunnel: [w179] -> w70
    tunnel: [w178] -> w69
    frame #0 {
      n68 = local read "Ic parameters"() -> (w183:T4)
      n69 = Unbundle By Name(w183) -> ("Records Num"=w182:i32, "Record Samples"=w181:u32)
      n70 = shared-variable-write(w186, w185, w183) -> (w184:refnum<k21>, w179:errorcluster)  [unwired: 1 in, 1 out]
      n71 = To Long Integer(number=w181) -> (32bit integer=w180:i32)
      n72 = Multiply(x=w182, y=w180) -> (x*y=w178:i32)
    }
  }
  n73 = local read "PCreaderI"() -> (w10:refnum<k21>)
  n74 = call "network stream read bulk.vi"("endpoint in"=w10, "Data num"=w69, "error in (no error)"=w70) -> ("endpoint out"=w72:refnum<k21>, "Data"=w71:fxp<+/-,17,5>[], "error out"=w50:errorcluster)  [unwired: 5 in]
  n75 = To Double Precision Float(number=w71) -> (double precision float=w83:dbl[])
  n76 = for {
    tunnel: w83 -> [w188] mode=indexing
    tunnel: w82 -> [w194]
    shift-right: [w190] -> w48
    shift-left: dbl[] [] -> [w189]
    i -> [w193]
    n77 = Quotient & Remainder(x=w193, y=w194) -> (x-y*floor(x/y)=w192:i32)  [unwired: 1 out]
    n78 = Equal?(x="Read point", y=w192) -> (x = y?=w187:bool)
    n79 = case shown="True" w187 {
      tunnel: [w195 w198] -> w190
      tunnel: w189 -> [w195 w197]
      tunnel: w188 -> [_ w196]
      frame False {
      }
      frame True {
        n80 = Build Array (concatenate)(w197, w196) -> (w198:dbl[])
      }
    }
  }
  "Array" <- w48
  n81 = call "datatofile 1c.vi"("A1"=w48, "error in"=w50, "title"="", "file path (dialog if empty)"=w53) -> ("error out"=w49:errorcluster)  [unwired: 7 in]
  n82 = call <vilib>:"Histogram.vi"("intervals"=100, "X"=w48) -> ("Histogram Graph"=→"Histogram Graph":T1)  [unwired: 6 in, 3 out]
  n83 = Destroy Stream Endpoint(8:w49, 11:w88) -> (0:w95:errorcluster)
  n84 = Destroy Stream Endpoint(8:w95, 11:w72) -> (0:w94:errorcluster)
  n85 = Destroy Stream Endpoint(8:w94, 11:w75) -> (0:w93:errorcluster)
  n86 = flat-sequence {
    tunnel: [w200] -> w9
    tunnel: w93 -> [w201]
    frame #0 {
      n87 = call "set RT Stop.vi"("error in (no error)"=w201, "RT Stop"=TRUE) -> ("error out"=w200:errorcluster)  [unwired: 9 in]
      n88 = local write "Done"(TRUE ("Done")) -> ()
    }
  }
  n89 = flat-sequence {
    tunnel: w9 -> [w207]
    tunnel: [w206] -> w8
    frame #0 {
      n90 = local read "DAQ_CMD_Writer endpoint"() -> (w205:refnum<k21>)
      n91 = local read "DAQ_AI_Reader endpoint"() -> (w203:refnum<k21>)
      n92 = call "RT simple command.vi"("Command"="Stop_DAQ1", "error in (no error)"=w207, "DAQ_CMD_Writer endpoint"=w205) -> ("error out"=w209:errorcluster, "DAQ_CMD_Writer endpoint out"=w204:refnum<k21>)  [unwired: 7 in]
      n93 = call "Stop cRIO DAQ.vi"("DAQ_AI_Reader endpoint"=w203, "DAQ_CMD_Writer endpoint"=w204, "error in (no error)"=w209) -> ("error out"=w206:errorcluster)  [unwired: 8 in]
    }
  }
  "error out" <- w8
